vi "LAB_VIWE_STACKEDSEQUENCE.vi"() -> ()   [LabVIEW 2020]
panel:
  out "x^2":dbl
  in  "NUM2":dbl
  in  "NUM1":dbl
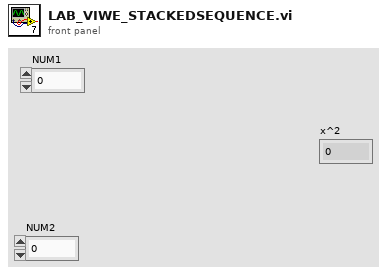
[diagram p1: front panel]
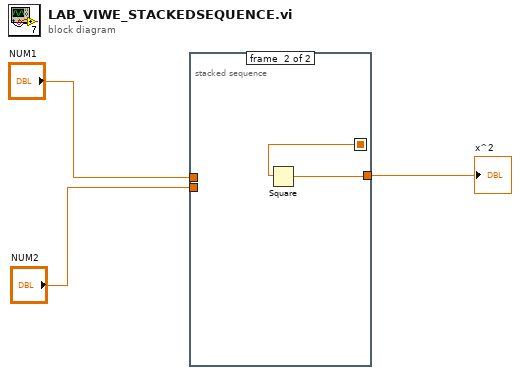
[diagram p0: block diagram]
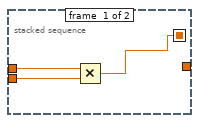
[diagram p2: hidden frame]
diagram:
  n1 = stacked-sequence {
    seq-local: [w4 _] -> [_ w8]
    tunnel: "NUM1" -> [w6 _]
    tunnel: "NUM2" -> [w5 _]
    tunnel: [_ w7] -> w1
    frame #0 {
      n2 = Multiply(x=w6, y=w5) -> (x*y=w4:dbl)
    }
    frame #1 {
      n3 = Square(x=w8) -> (x^2=w7:dbl)
    }
  }
  "x^2" <- w1
